vi "resistanceCalculator_RS485.vi"(0 "VISA resource name":refnum<visa-resource-name>, 1 "MIn":dbl=15.0, 2 "Max":dbl, 3 "Gear":dbl format="%#_13g", 4 "Incline":dbl, 5 "error in (no error)":errorcluster, 6 "Gear Max":dbl, 7 "kgs":dbl=83.91, 8 "Mod":bool) -> (9 "lbs":dbl, 12 "continuousADC":dbl, 13 "resistance":cluster{dbl, dbl}(graph), 14 "Result":dbl, 15 "Variable":dbl, 16 "DAC":dbl, 17 "Voltage":dbl, 18 "Difference":dbl, 19 "error out":errorcluster)   [LabVIEW 2018]
uses:
  <vilib>/express/express arith-compare/Formula/XNode/ExpressFormulaBlockNode.xnode
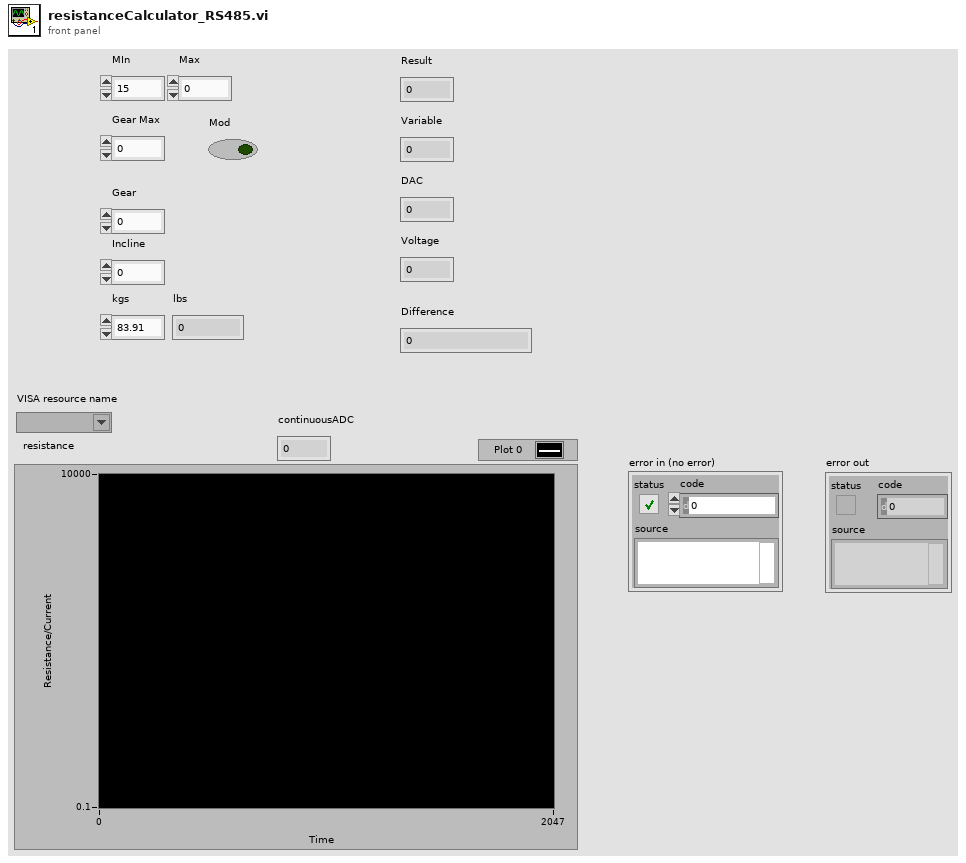
[diagram p1: front panel]
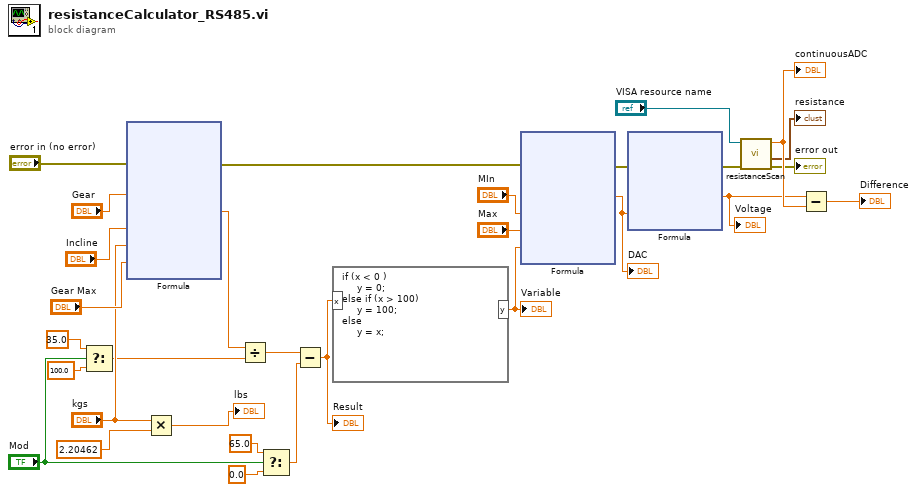
[diagram p0: block diagram]
diagram:
  n1 = Select(t=35.0 ("x"), s="Mod", f=100.0) -> (s? t:f=w11:dbl)
  n2 = xnode "Formula"("X1"="Gear", "X2"="Incline", "X3"="kgs", "X4"="Gear Max", "error in (no error)"="error in (no error)") -> ("Result"=w10:dbl, "error out"=w5:errorcluster)
  n3 = Multiply(x="kgs", y=2.20462) -> (x*y=→"lbs":dbl)
  n4 = Divide(x=w10, y=w11) -> (x/y=w7:dbl)
  n5 = Select(t=65.0 ("y"), s="Mod", f=0.0) -> (s? t:f=w8:dbl)
  n6 = Subtract(x=w7, y=w8) -> (x-y=w16:dbl)
  "Result" <- w16
  n7 = formula code="if (x < 0 )\n     y = 0;\nelse if (x > 100)\n     y = 100;\nelse\n     y = x;"("x"=w16) -> ("y"=w17:dbl)
  "Variable" <- w17
  n8 = xnode "Formula"("Min"="MIn", "Max"="Max", "Vin"=w17, "error in (no error)"=w5) -> ("Result"=w18:dbl, "error out"=w4:errorcluster)
  "DAC" <- w18
  n9 = xnode "Formula"("Din"=w18, "error in (no error)"=w4) -> ("Result"=w19:dbl, "error out"=w3:errorcluster)
  "Voltage" <- w19
  n10 = call "resistanceScan.vi"("error in (no error)"=w3, "VISA Refnum in"="VISA resource name") -> ("error out"=→"error out":errorcluster, "RESISTANCE/CURRENT"=→"resistance":cluster{dbl, dbl}, "ADC value"=w22:dbl)  [unwired: 5 in, 2 out]
  "continuousADC" <- w22
  n11 = Subtract(x=w19, y=w22) -> (x-y=→"Difference":dbl)
